vi "3_2_(2).vi"() -> ()   [LabVIEW 2012]
uses:
  Control 1.ctl
  Global 1.vi
panel:
  in  "Таблиця 1 - Вхідні дані":string[][](table)
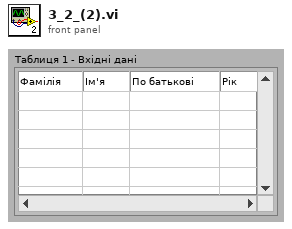
[diagram p1: front panel]
types:
  T1 = typedef "Control 1.ctl" = enum16{"Серверу", "Клієнту", "Зчитати", "Стоп", "1", "2", "3", "4"}
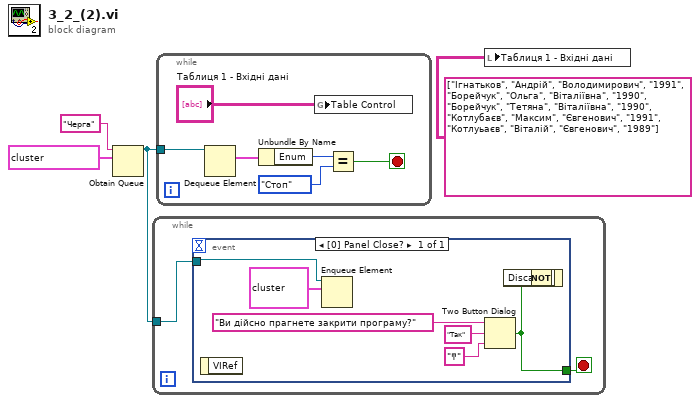
[diagram p0: block diagram]
diagram:
  n1 = Obtain Queue(name (unnamed)="Черга", element data type=cluster{"variant":variant, "Enum":T1} {"variant"=variant, "Enum"=enum."Стоп"}) -> (queue out=w2:refnum<queue>)  [unwired: 3 in, 2 out]
  n2 = while {
    tunnel: w2 -> [w5]
    stop <- w6 stop-if-true
    n3 = event shown="[0] Panel Close?" {
      selector: _ -> [_]
      dyn-events: _ -> [_]
      timeout: _ -> [_]
      tunnel: [w9] -> w6
      tunnel: w5 -> [w8]
      event Panel Close? {
        n4 = event-data() -> ()  [unwired: 1 in, 1 out]
        n5 = Enqueue Element(queue=w8, element=cluster{"variant":variant, "Enum":T1} {"variant"=variant, "Enum"=enum."Стоп"}) -> ()  [unwired: 2 in, 3 out]
        n6 = Two Button Dialog(message="Ви дійсно прагнете закрити програму?", 1:"ͳ" ("F button name (\"Cancel\")"), 2:"Так" ("T button name (\"OK\")")) -> (T button?=w9:bool)
        n7 = Not(x=w9) -> (.not. x?=w10:bool)
        n8 = event-data("Discard?"=w10) -> ()  [unwired: 1 in, 1 out]
      }
    }
  }
  n9 = while {
    tunnel: w2 -> [w19]
    stop <- w16 stop-if-true
    n10 = Dequeue Element(queue=w19) -> (element=w18:cluster{"variant":variant, "Enum":T1})  [unwired: 2 in, 3 out]
    n11 = Unbundle By Name(w18) -> ("Enum"=w15:T1)
    n12 = global write "Global 1.vi" "Table Control"("Таблиця 1 - Вхідні дані") -> ()
    n13 = Equal?(x=w15, y=Control_1."Стоп" ("Enum")) -> (x = y?=w16:bool)
  }
  n14 = local write "Таблиця 1 - Вхідні дані"(string[][] [["Ігнатьков", "Андрій", "Володимирович", "1991"], ["Борейчук", "Ольга", "Віталіївна", "1990"], ["Борейчук", "Тетяна", "Віталіївна", "1990"], ["Котлубаєв", "Максим", "Євгенович", "1991"], ["Котлуьаєв", "Віталій", "Євгенович", "1989"]] ("Таблиця 1")) -> ()
